vi "LVMark_Find_General_Match.vi"(7 "optype":T2, 8 "error in":errorcluster, 9 "Operations":T1[](array[typedef]), 10 "regular expression":string="(\\*\\*|__|\\[bold\\])(?=\\S)(.+?)(?<=\\S)\\1", 11 "ML string":string) -> (0 "error out":errorcluster, 1 "Operations out":T1[](array[typedef]), 3 "ML string out":string)   [LabVIEW 2009]
doc: "Add any of the found elements to the list of operations that will be performed on the text control."
uses:
  LVMark_opcluster.ctl
  LVMark_optype.ctl
  <vilib>/regexp/Match Regular Expression.xnode
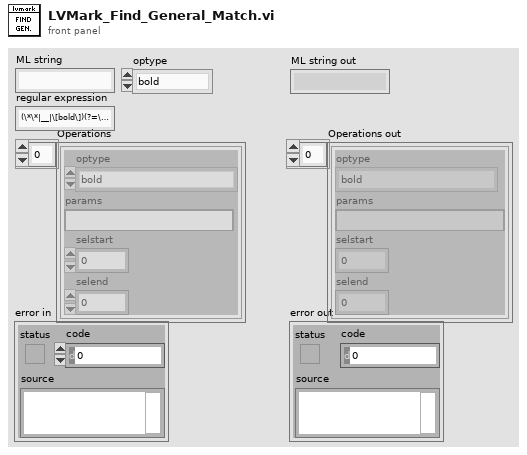
[diagram p1: front panel]
types:
  T1 = typedef "LVMark_opcluster.ctl" = cluster{"optype":T2, "params":string, "selstart":i32, "selend":i32}
  T2 = typedef "LVMark_optype.ctl" = enum16{"bold", "italic", "underline", "color", "font", "fontsize", "strikethrough"}
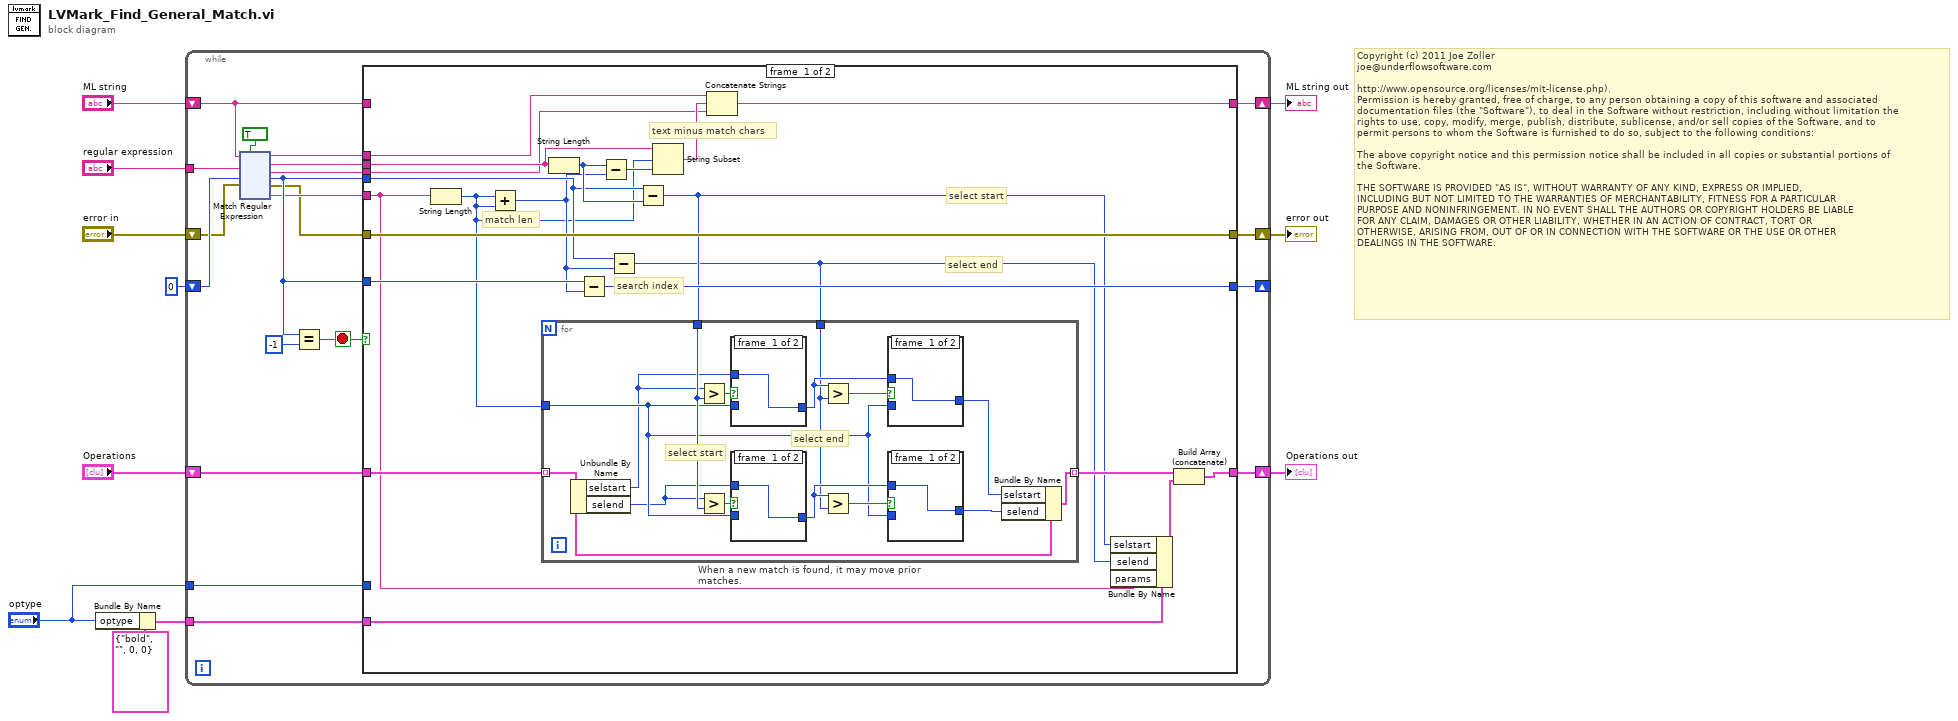
[diagram p0: block diagram]
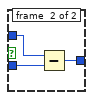
[diagram p2: hidden frame]
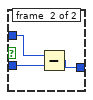
[diagram p3: hidden frame]
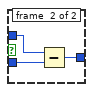
[diagram p4: hidden frame]
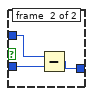
[diagram p5: hidden frame]
diagram:
  # "Copyright (c) 2011 Joe Zoller\njoe@underflowsoftware.com\n\nhttp://www.opensource.org/licenses/mit-license.php).\nPermission is hereby granted, free of charge, to any person obtaining a copy of this software and associated\ndocumentation files (the \"Software\"), to deal in the Software without restriction, including without limitation the\nrights to use, copy, modify, merge, publish, distribute, sublicense, and/or sell copies of the Software, and to\npermit persons to whom the Software is furnished to do so, subject to the following conditions:\n\nThe above copyright notice and this permission notice shall be included in all copies or substantial portions of\nthe Software.\n\nTHE SOFTWARE IS PROVIDED \"AS IS\", WITHOUT WARRANTY OF ANY KIND, EXPRESS OR IMPLIED,\nINCLUDING BUT NOT LIMITED TO THE WARRANTIES OF MERCHANTABILITY, FITNESS FOR A PARTICULAR\nPURPOSE AND NONINFRINGEMENT. IN NO EVENT SHALL THE AUTHORS OR COPYRIGHT HOLDERS BE LIABLE\nFOR ANY CLAIM, DAMAGES OR OTHER LIABILITY, WHETHER IN AN ACTION OF CONTRACT, TORT OR\nOTHERWISE, ARISING FROM, OUT OF OR IN CONNECTION WITH THE SOFTWARE OR THE USE OR OTHER\nDEALINGS IN THE SOFTWARE."
  n1 = Bundle By Name(cluster=T1 {"optype"=enum."bold", "params"="", "selstart"=0, "selend"=0} ("operation"), "optype"="optype") -> (w3:T1)
  n2 = while {
    shift-right: [w23] -> w7
    shift-left: "ML string" -> [w30]
    shift-right: [w25] -> w6
    shift-left: "error in" -> [w17]
    shift-right: [w21] -> _
    shift-left: 0 -> [w24]
    shift-right: [w19] -> w2
    shift-left: "Operations" -> [w20]
    tunnel: "regular expression" -> [w15]
    tunnel: w3 -> [w14]
    tunnel: "optype" -> [w13]
    stop <- w26 stop-if-true
    n3 = xnode "Match Regular Expression"("input string"=w30, "regular expression"=w15, "offset (0)"=w24, "error in"=w17, "ignore case? (F)"=TRUE) -> ("before match"=w29:string, "whole match"=w28:string, "after match"=w27:string, "offset past match"=w22:i32, "error out"=w16:errorcluster, "submatch 1"=w18:string)  [unwired: 1 in]
    n4 = Equal?(x=w22, y=-1) -> (x = y?=w26:bool)
    n5 = case shown="False" w26 {
      tunnel: w30 -> [_ w196]
      tunnel: [w160 w196] -> w23
      tunnel: w29 -> [w159 _]
      tunnel: w28 -> [w158 _]
      tunnel: w27 -> [w157 _]
      tunnel: w22 -> [w153 _]
      tunnel: w16 -> [w154 w195]
      tunnel: [w154 w195] -> w25
      tunnel: w22 -> [w152 w194]
      tunnel: [w151 w194] -> w21
      tunnel: w20 -> [w147 w193]
      tunnel: [w150 w193] -> w19
      tunnel: w18 -> [w142 _]
      tunnel: w14 -> [w141 _]
      tunnel: w13 -> [_ _]
      frame #0 {
        # "text minus match chars"
        # "search index"
        # "match len"
        # "select start"
        # "select end"
        n6 = String Length(string=w142) -> (length=w148:i32)
        n7 = Add(x=w148, y=w148) -> (x+y=w149:i32)
        n8 = String Length(string=w158) -> (length=w155:i32)
        n9 = Subtract(x=w152, y=w149) -> (x-y=w151:i32)
        n10 = Subtract(x=w155, y=w149) -> (x-y=w156:i32)
        n11 = Subtract(x=w153, y=w149) -> (x-y=w144:i32)
        n12 = Subtract(x=w153, y=w155) -> (x-y=w145:i32)
        n13 = for "When a new match is found, it may move prior matches." {
          tunnel: w145 -> [w170]
          tunnel: w148 -> [w169]
          tunnel: w144 -> [w168]
          tunnel: w147 -> [w165] mode=indexing
          tunnel: [w162] -> w146 mode=indexing
          # "select start"
          # "select end"
          n14 = Unbundle By Name(w165) -> ("selstart"=w167:i32, "selend"=w166:i32)
          n15 = Greater?(x=w167, y=w170) -> (0:w176:bool)
          n16 = Greater?(x=w166, y=w170) -> (0:w171:bool)
          n17 = case shown="True" w176 {
            tunnel: w167 -> [w189 w192]
            tunnel: w169 -> [_ w191]
            tunnel: [w189 w190] -> w174
            frame #0 {
            }
            frame #1 {
              n18 = Subtract(x=w192, y=w191) -> (x-y=w190:i32)
            }
          }
          n19 = case shown="True" w171 {
            tunnel: w166 -> [w181 w184]
            tunnel: w169 -> [_ w183]
            tunnel: [w181 w182] -> w173
            frame #0 {
            }
            frame #1 {
              n20 = Subtract(x=w184, y=w183) -> (x-y=w182:i32)
            }
          }
          n21 = Greater?(x=w174, y=w168) -> (0:w175:bool)
          n22 = Greater?(x=w173, y=w168) -> (0:w172:bool)
          n23 = case shown="True" w175 {
            tunnel: w174 -> [w185 w188]
            tunnel: w169 -> [_ w187]
            tunnel: [w185 w186] -> w164
            frame #0 {
            }
            frame #1 {
              n24 = Subtract(x=w188, y=w187) -> (x-y=w186:i32)
            }
          }
          n25 = case shown="True" w172 {
            tunnel: w173 -> [w177 w180]
            tunnel: w169 -> [_ w179]
            tunnel: [w177 w178] -> w163
            frame #0 {
            }
            frame #1 {
              n26 = Subtract(x=w180, y=w179) -> (x-y=w178:i32)
            }
          }
          n27 = Bundle By Name(cluster=w165, "selstart"=w164, "selend"=w163) -> (w162:T1)
        }
        n28 = String Subset(string=w158, offset (0)=w148, length (rest)=w156) -> (substring=w161:string)
        n29 = Concatenate Strings(w159, w161, w157) -> (w160:string)
        n30 = Bundle By Name(cluster=w141, "selstart"=w145, "selend"=w144, "params"=w142) -> (w143:T1)
        n31 = Build Array (concatenate)(w146, w143) -> (w150:T1[])
      }
      frame #1 {
      }
    }
  }
  "ML string out" <- w7
  "error out" <- w6
  "Operations out" <- w2
